vi "symmetry_transform_to_marginal_destructive.vi"(4 "ROI (x,y,w,h)":i32[](array[numeric]), 5 "margin":i32=15, 6 "Transform Columns?":bool, 7 "LineWidth(Pixels)":i32, 8 "Pixel Pointer":u64 format="%.0x") -> (2 "Marginal":sgl[](array[numeric]), 3 "Pixel Pointer out":u64 format="%.0x")   [LabVIEW 2010]
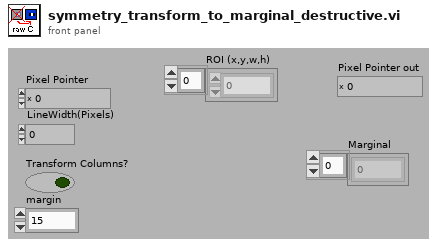
[diagram p1: front panel]
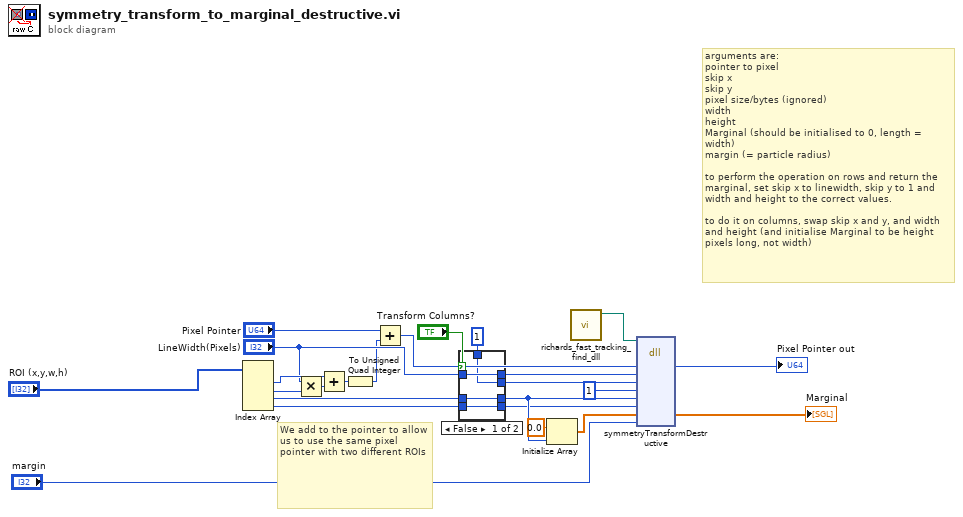
[diagram p0: block diagram]
diagram:
  # "We add to the pointer to allow us to use the same pixel pointer with two different ROIs"
  # "arguments are:\npointer to pixel\nskip x \nskip y\npixel size/bytes (ignored)\nwidth\nheight\nMarginal (should be initialised to 0, length = width)\nmargin (= particle radius)\n\nto perform the operation on rows and return the marginal, set skip x to linewidth, skip y to 1 and width and height to the correct values.\n\nto do it on columns, swap skip x and y, and width and height (and initialise Marginal to be height pixels long, not width)"
  n1 = Index Array(array="ROI (x,y,w,h)") -> (element #1=w17:i32, element #2=w19:i32, element #3=w5:i32, element #4=w22:i32)  [unwired: 4 in]
  n2 = Multiply(x="LineWidth(Pixels)", y=w19) -> (x*y=w18:i32)
  n3 = Add(x=w17, y=w18) -> (x+y=w15:i32)
  n4 = To Unsigned Quad Integer(1:w15) -> (0:w14:u64)
  n5 = Add(x="Pixel Pointer", y=w14) -> (x+y=w13:u64)
  n6 = case shown="False" "Transform Columns?" {
    tunnel: [w28 w32] -> w12
    tunnel: 1 ("LineWidth(Pixels)") -> [w27 w32]
    tunnel: [w27 w31] -> w11
    tunnel: "LineWidth(Pixels)" -> [w28 w31]
    tunnel: [w26 w29] -> w10
    tunnel: [w25 w30] -> w9
    tunnel: w5 -> [w26 w30]
    tunnel: w22 -> [w25 w29]
    frame False {
    }
    frame True {
    }
  }
  n7 = Initialize Array(sgl 0.0 ("element"), w10) -> (w3:sgl[])
  n8 = call "richards_fast_tracking_find_dll.vi"() -> ("appended path"=w1:path)  [unwired: 11 in]
  n9 = dll-call lib="C:/Users/alinnenberger/Desktop/Cube/red_tweezers_1_4_rc0/RichardFastTracking/symmetrytransform32.dll" fn="symmetryTransformDestructive"(path in=w1, "pixelPointer"=w13, "skipx"=w12, "skipy"=w11, "pixelSizeInBytes"=1 ("LineWidth(Pixels)"), "width"=w10, "height"=w9, "xMarginal"=w3, "radius"="margin") -> ("pixelPointer"=→"Pixel Pointer out":u64, "xMarginal"=→"Marginal":sgl[])  [unwired: 9 in, 2 out]
